vi "Create Oasis authorization file.vi"(5 "selected path":path, 6 "CORE Options":T1={"CORE"=TRUE, "Emitter Manager"=TRUE, "Interference Manager"=TRUE, "FCC Database"=TRUE, "Scheduler"=TRUE, "Drive Test"=TRUE, "TBD Option 3"=FALSE, "TBD Option 4"=FALSE, "US Map"=TRUE, "Europe Map"=FALSE, "China Map"=FALSE, "Africa"=FALSE, "North-South America"=FALSE, "10 Drivers"=FALSE, "25 Drivers"=FALSE, "50 Drivers"=FALSE, "Advantest"=FALSE, "Agilent"=TRUE, "Future"=FALSE, "Anritsu"=TRUE, "Future"=FALSE, "Future"=FALSE, "Rohde & Schwarz"=TRUE, "Spectrum Analyzer Simulator"=TRUE, "Willtek 9100"=FALSE, "NetTek"=FALSE, "NI 5660"=FALSE, "Future"=FALSE, "ICOM"=FALSE, "Future"=FALSE, "Future"=FALSE, "Future"=FALSE}, 7 "USE USB  KEY?":bool, 8 "error in (no error)":errorcluster, 9 "Expire Date":timestamp=timestamp(3413740012.677496 s since 1904-01-01), 10 "oasis authorization key":string="1", 11 "user machine site code":string="1818747070") -> (0 "error out":errorcluster, 1 "Log String":string, 2 "HW ID":string)   [LabVIEW 2011]
uses:
  CORE Options.ctt
  Authorization XML.ctl
panel:
  out "Path":path
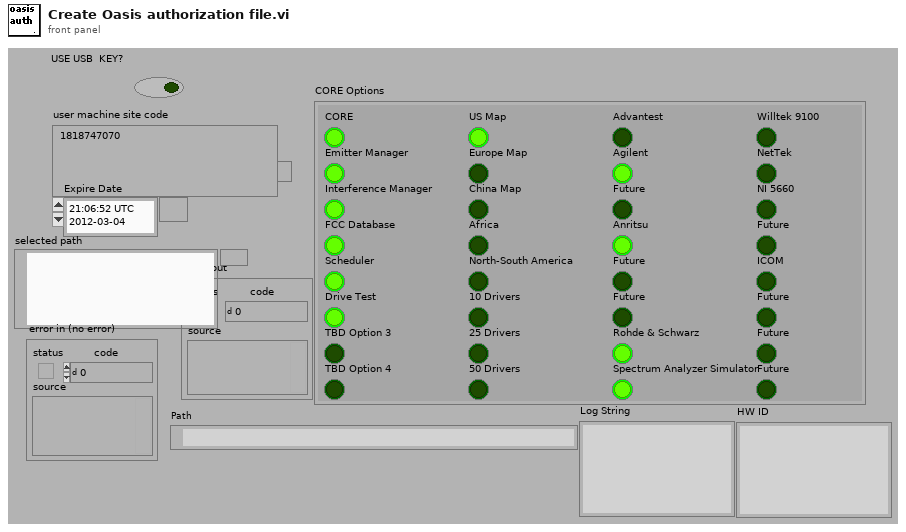
[diagram p1: front panel]
types:
  T1 = typedef "CORE Options.ctt" = cluster{"CORE":bool, "Emitter Manager":bool, "Interference Manager":bool, "FCC Database":bool, "Scheduler":bool, "Drive Test":bool, "TBD Option 3":bool, "TBD Option 4":bool, "US Map":bool, "Europe Map":bool, "China Map":bool, "Africa":bool, "North-South America":bool, "10 Drivers":bool, "25 Drivers":bool, "50 Drivers":bool, "Advantest":bool, "Agilent":bool, "Future":bool, "Anritsu":bool, "Future":bool, "Future":bool, "Rohde & Schwarz":bool, "Spectrum Analyzer Simulator":bool, "Willtek 9100":bool, "NetTek":bool, "NI 5660":bool, "Future":bool, "ICOM":bool, "Future":bool, "Future":bool, "Future":bool}
  T2 = typedef "Authorization XML.ctl" = cluster{"Hardware ID":string, "oasis Serial Number":string, "Feature":cluster{"#attributes":cluster{"Name":string, "Value":string}}[], "valid":bool, "Expire Date":dbl}
  T3 = cluster{"#attributes":cluster{"Name":string, "Value":string}}[]
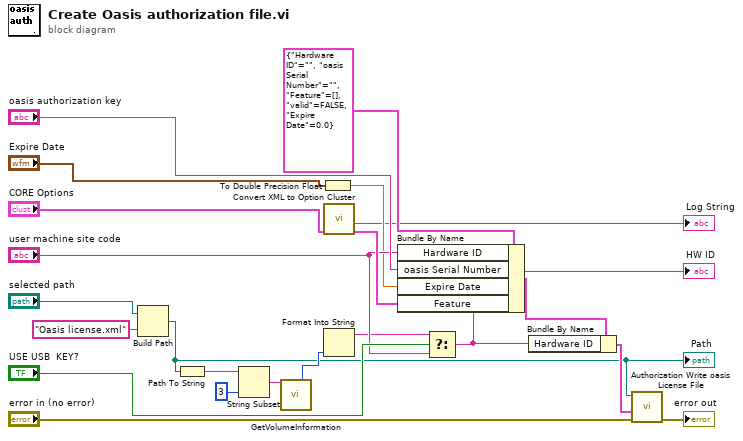
[diagram p0: block diagram]
diagram:
  n1 = Build Path(base path="selected path", name or relative path="Oasis license.xml" ("default name")) -> (appended path=w4:path)
  "Path" <- w4
  n2 = Path To String(path=w4) -> (string=w10:string)
  n3 = String Subset(string=w10, length (rest)=3 ("length (rest)")) -> (substring=w8:string)  [unwired: 1 in]
  n4 = call "GetVolumeInformation.vi"("RootPathName (C:\\)"=w8) -> ("VolumeSerialNumber"=w11:u32)  [unwired: 8 in, 6 out]
  n5 = To Double Precision Float(number="Expire Date") -> (double precision float=w12:dbl)
  n6 = call "Convert XML to Option Cluster.vi"("CORE Options 2"="CORE Options") -> ("Feature 2"=w18:T3, "String"=→"Log String":string)  [unwired: 8 in, 1 out]
  n7 = Format Into String(w11) -> (resulting string=w6:string)  [unwired: 3 in, 1 out]
  n8 = Bundle By Name(cluster=T2 {"Hardware ID"="", "oasis Serial Number"="", "Feature"=[], "valid"=FALSE, "Expire Date"=0.0} ("Authorization"), "Hardware ID"="user machine site code", "oasis Serial Number"="oasis authorization key", "Expire Date"=w12, "Feature"=w18) -> (w16:T2)
  n9 = Select(t=w6, s="USE USB  KEY?", f="user machine site code") -> (s? t:f=w1:string)
  "HW ID" <- w1
  n10 = Bundle By Name(cluster=w16, "Hardware ID"=w1) -> (w7:T2)
  n11 = call "Authorization Write oasis License File.vi"("error in (no error)"="error in (no error)", "Authorization"=w7, "Path"=w4) -> ("error out"=→"error out":errorcluster)  [unwired: 8 in]
